vi "main.vi"() -> ()   [LabVIEW 2023]
uses:
  <vilib>/Utility/file.llb/Write Delimited Spreadsheet (DBL).vi
  <vilib>/Utility/file.llb/Read Delimited Spreadsheet (DBL).vi
  <vilib>/Instr/_visa.llb/VISA Configure Serial Port (Instr).vi
panel:
  in  "Threshold":dbl=2000.0
  in  "Open Button":bool
  in  "Save Button":bool
  out "X max":dbl
  out "X min":dbl
  out "Y max":dbl
  out "Y min":dbl
  out "Z max":dbl
  out "Z min":dbl
  out "Acc":cluster{dbl[], dbl[]}[](graph) caption="XY Graph - Dark"
  out "Z max":dbl
  out "Z min":dbl
  out "Y max":dbl
  out "Y min":dbl
  out "X min":dbl
  out "X max":dbl
  in  "Delete":bool
  out "Mag":cluster{dbl[], dbl[]}[](graph) caption="XY Graph - Dark"
  in  "Button":bool
  out "Raw Data":string
  in  "timeout (ms)":u32=100
  in  "term. char (0xA = '\\n' = LF)":u8=10 format="%.0x"
  in  "baud rate":u32=9600
  in  "COM PORT":refnum<visa-resource-name>
  # "Mag"
  # "Acc"
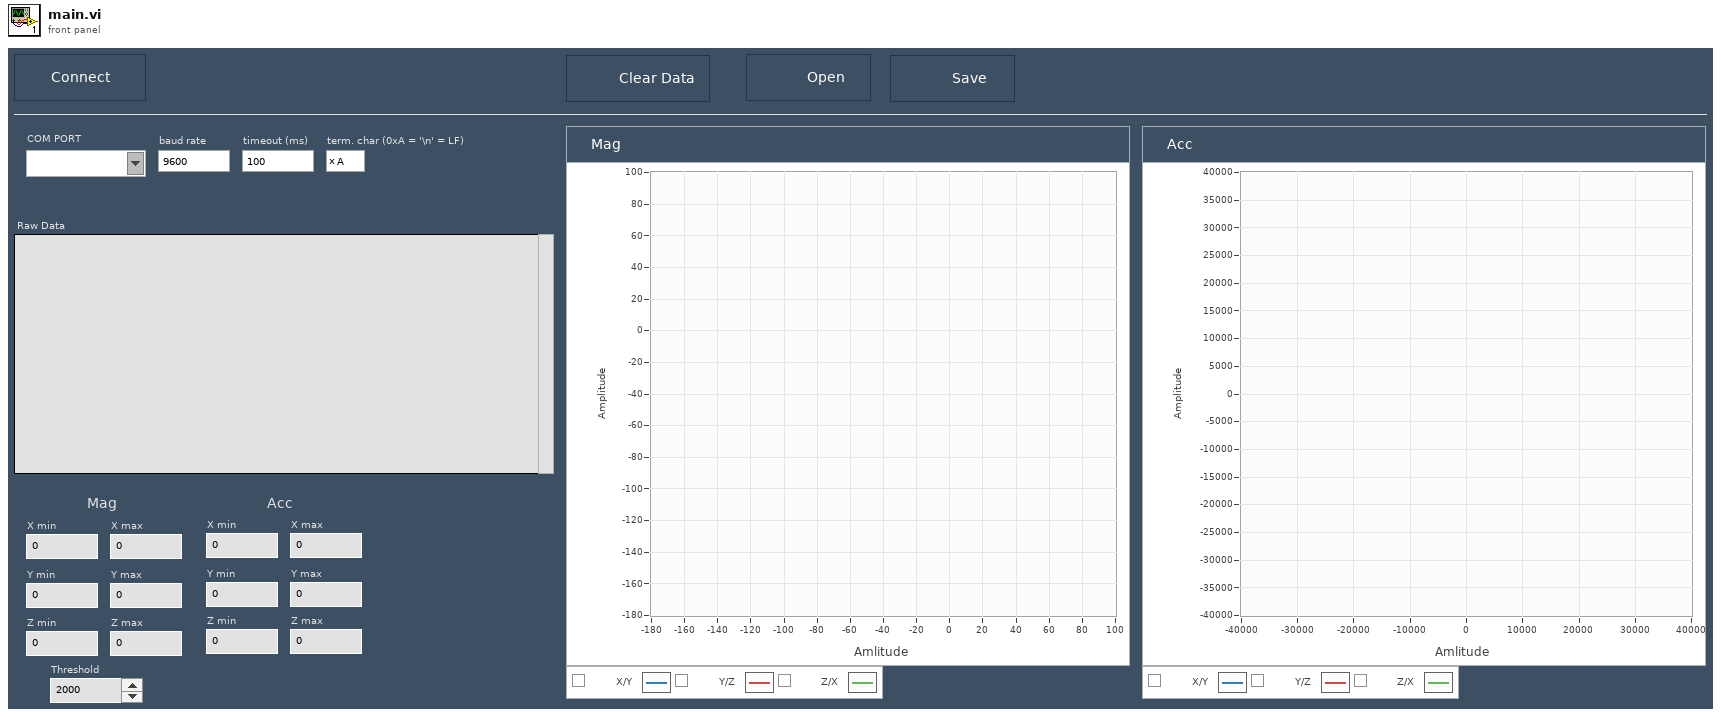
[diagram p1: front panel]
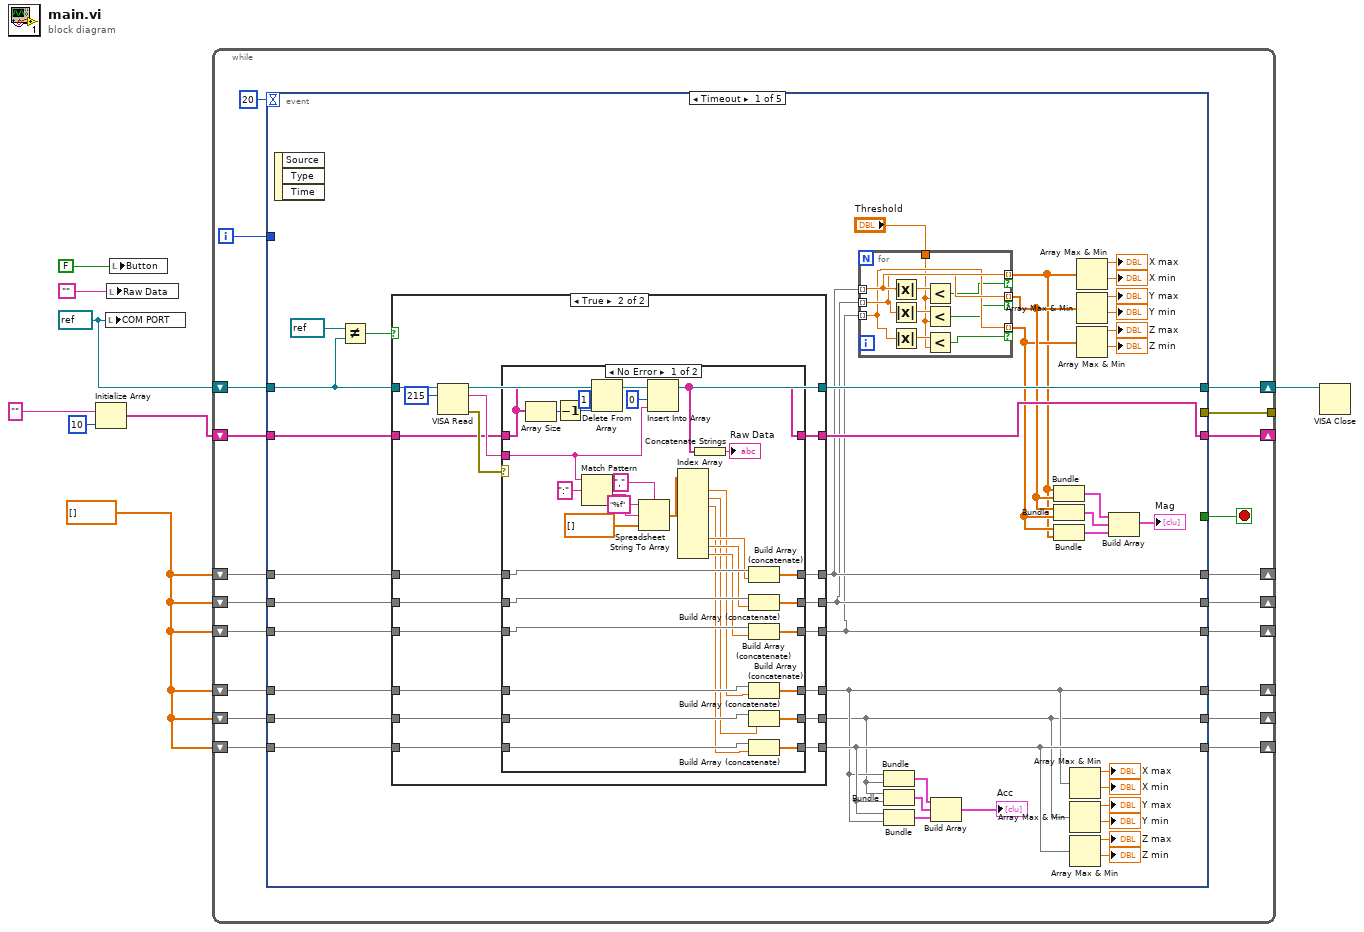
[diagram p0: block diagram]
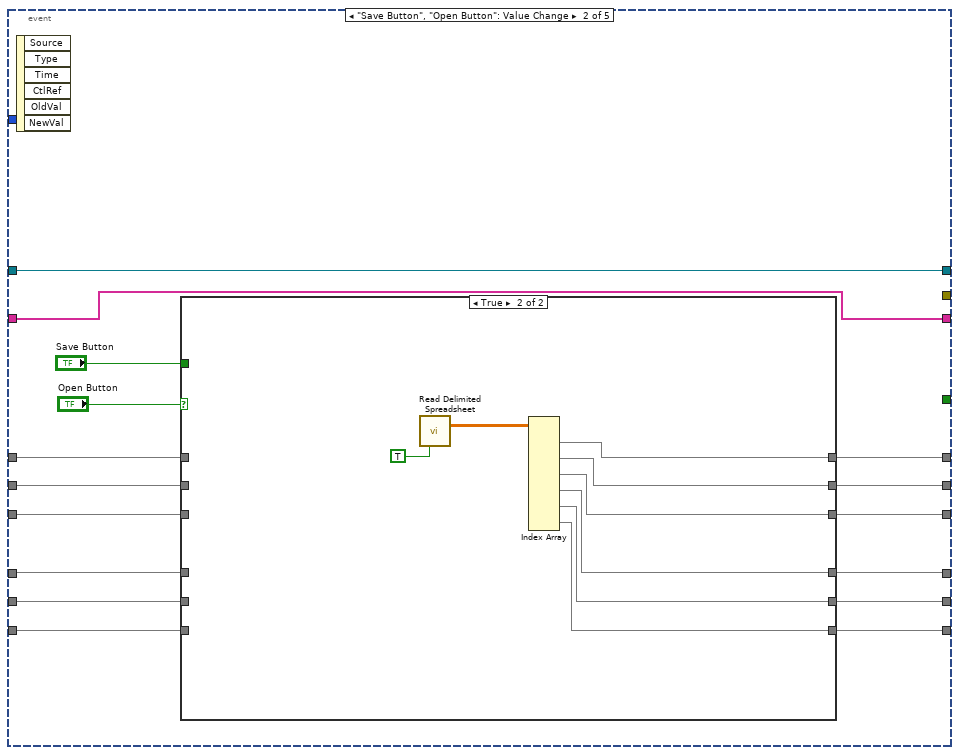
[diagram p4: hidden frame]
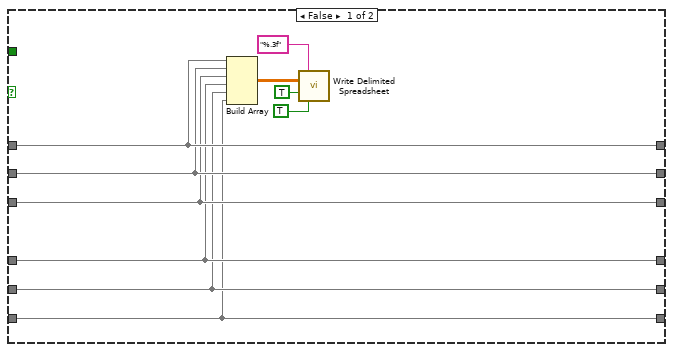
[diagram p5: hidden frame]
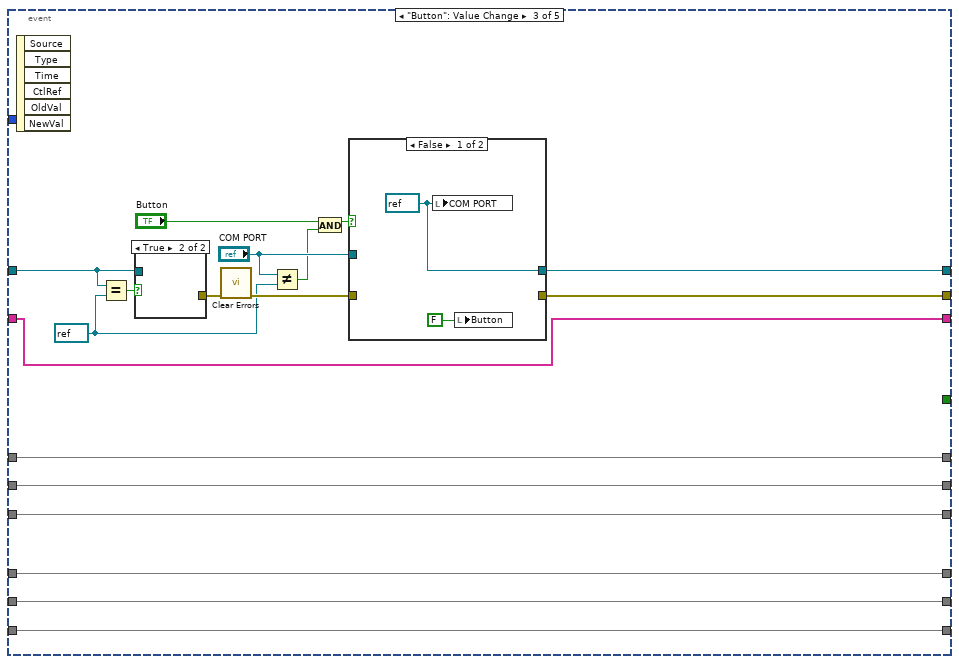
[diagram p6: hidden frame]
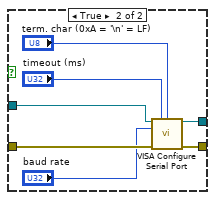
[diagram p7: hidden frame]
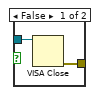
[diagram p8: hidden frame]
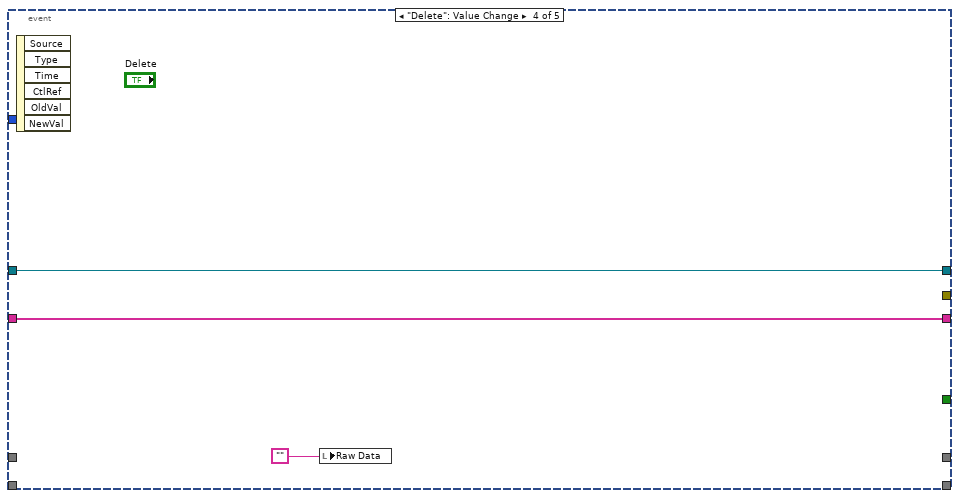
[diagram p9: hidden frame]
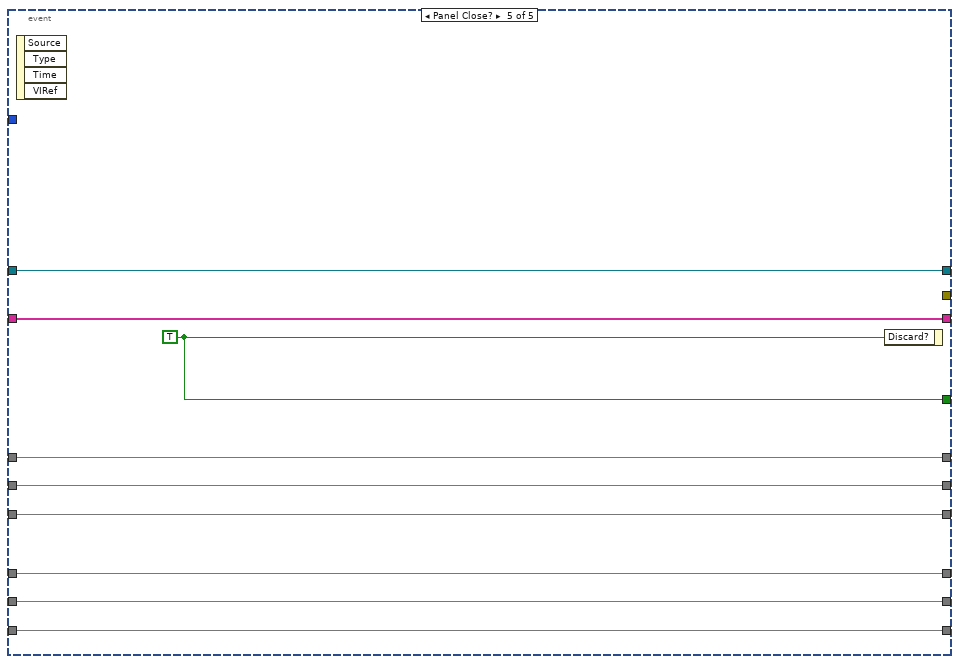
[diagram p10: hidden frame]
diagram:
  w5 = dbl[] [] ("array")
  w7 = refnum<visa-resource-name> refnum ("COM PORT")
  n1 = Initialize Array("", 10 ("dimension size")) -> (w1:string[])
  n2 = local write "COM PORT"(w7) -> ()
  n3 = local write "Raw Data"("") -> ()
  n4 = local write "Button"(FALSE ("connect")) -> ()
  n5 = while {
    tunnel: [w28] -> _
    shift-right: [w27] -> w8
    shift-left: w7 -> [w26]
    shift-right: [w23] -> _
    shift-left: w5 -> [w22]
    shift-right: [w21] -> _
    shift-left: w5 -> [w20]
    shift-right: [w19] -> _
    shift-left: w5 -> [w18]
    shift-right: [w14] -> _
    shift-left: w5 -> [w15]
    shift-right: [w13] -> _
    shift-left: w5 -> [w16]
    shift-right: [w12] -> _
    shift-left: w5 -> [w17]
    shift-right: [w10] -> _
    shift-left: w1 -> [w9]
    i -> [w11]
    stop <- w25 stop-if-true
    n6 = event shown="[0] Timeout" {
      selector: _ -> [_ _ _ _ _]
      dyn-events: _ -> [_ _ _ _ _]
      timeout: 20 -> [_ _ _ _ _]
      tunnel: [_ _ w196 _ _] -> w28
      tunnel: [w70 w163 w195 w213 w222] -> w27
      tunnel: w26 -> [w43 w163 w191 w213 w222]
      tunnel: [_ _ _ _ w221] -> w25
      tunnel: [w35 w160 w194 _ w220] -> w23
      tunnel: w22 -> [w69 w159 w194 _ w220]
      tunnel: [w34 w158 w193 _ w219] -> w21
      tunnel: w20 -> [w68 w157 w193 _ w219]
      tunnel: [w33 w155 w192 _ w218] -> w19
      tunnel: w18 -> [w67 w156 w192 _ w218]
      tunnel: w15 -> [w58 w153 w189 _ w217]
      tunnel: w16 -> [w59 w152 w188 _ w216]
      tunnel: w17 -> [w60 w149 w187 _ w215]
      tunnel: [w39 w154 w189 _ w217] -> w14
      tunnel: [w38 w151 w188 _ w216] -> w13
      tunnel: [w40 w150 w187 _ w215] -> w12
      tunnel: w11 -> [_ _ _ _ _]
      tunnel: [w37 w148 w182 w211 w214] -> w10
      tunnel: w9 -> [w36 w148 w182 w211 w214]
      event Timeout {
        n7 = event-data() -> ()  [unwired: 1 in, 3 out]
        n8 = Not Equal?(x=refnum<visa-resource-name> refnum ("COM PORT"), y=w43) -> (x != y?=w41:bool)
        n9 = case shown="True" w41 {
          tunnel: [w88 w107] -> w70
          tunnel: w43 -> [w88 w103]
          tunnel: [w87 w101] -> w35
          tunnel: w69 -> [w87 w102]
          tunnel: [w86 w100] -> w34
          tunnel: w68 -> [w86 w99]
          tunnel: [w85 w98] -> w33
          tunnel: w67 -> [w85 w97]
          tunnel: w58 -> [w84 w94]
          tunnel: w59 -> [w83 w95]
          tunnel: w60 -> [w82 w96]
          tunnel: [w84 w93] -> w39
          tunnel: [w83 w92] -> w38
          tunnel: [w82 w91] -> w40
          tunnel: [w81 w90] -> w37
          tunnel: w36 -> [w81 w89]
          frame False {
          }
          frame True {
            n10 = VISA Read(VISA resource name=w103, byte count=u32 215) -> (VISA resource name out=w107:refnum<visa-resource-name>, read buffer=w105:string, error out=w104:errorcluster)  [unwired: 1 in, 1 out]
            n11 = case shown="No Error" w104 {
              tunnel: w105 -> [w110 _]
              tunnel: w102 -> [w135 w147]
              tunnel: [w126 w147] -> w101
              tunnel: [w128 w146] -> w100
              tunnel: w99 -> [w133 w146]
              tunnel: [w127 w145] -> w98
              tunnel: w97 -> [w132 w145]
              tunnel: w94 -> [w125 w142]
              tunnel: w95 -> [w124 w143]
              tunnel: w96 -> [w123 w144]
              tunnel: [w121 w142] -> w93
              tunnel: [w122 w143] -> w92
              tunnel: [w120 w144] -> w91
              tunnel: [w109 w141] -> w90
              tunnel: w89 -> [w116 w141]
              frame No Error {
                n12 = Array Size(array=w116) -> (size(s)=w115:i32)
                n13 = Decrement(x=w115) -> (x-1=w114:i32)
                n14 = Match Pattern(string=w110, regular expression=":") -> (after substring=w138:string)  [unwired: 1 in, 3 out]
                n15 = Delete From Array(array=w116, length=1, index=w114) -> (array with subset deleted=w112:string[])  [unwired: 1 out]
                n16 = Spreadsheet String To Array(delimiter (Tab)=",", format string="%f", spreadsheet string=w138, array type (2D Dbl)=dbl[] []) -> (array=w134:dbl[])
                n17 = Insert Into Array(array=w112, index=0, new element=w110) -> (w109:string[])
                n18 = Index Array(array=w134) -> (element #1=w119:dbl, element #2=w118:dbl, element #3=w117:dbl, element #7=w131:dbl, element #8=w130:dbl, element #9=w129:dbl)  [unwired: 9 in, 3 out]
                n19 = Concatenate Strings(w109) -> (→"Raw Data":string)
                n20 = Build Array (concatenate)(w135, w131) -> (w126:dbl[])
                n21 = Build Array (concatenate)(w133, w130) -> (w128:dbl[])
                n22 = Build Array (concatenate)(w132, w129) -> (w127:dbl[])
                n23 = Build Array (concatenate)(w125, w119) -> (w121:dbl[])
                n24 = Build Array (concatenate)(w124, w118) -> (w122:dbl[])
                n25 = Build Array (concatenate)(w123, w117) -> (w120:dbl[])
              }
              frame Error {
              }
            }
          }
        }
        n26 = for {
          tunnel: w35 -> [w77] mode=indexing
          tunnel: w34 -> [w76] mode=indexing
          tunnel: w33 -> [w75] mode=indexing
          tunnel: "Threshold" -> [w74]
          tunnel: [w77] -> w29 mode=indexing if=w72
          tunnel: [w76] -> w31 mode=indexing if=w73
          tunnel: [w75] -> w30 mode=indexing if=w71
          n27 = Absolute Value(x=w77) -> (abs(x)=w80:dbl)
          n28 = Absolute Value(x=w76) -> (abs(x)=w79:dbl)
          n29 = Absolute Value(x=w75) -> (abs(x)=w78:dbl)
          n30 = Less?(x=w80, y=w74) -> (x < y?=w72:bool)
          n31 = Less?(x=w79, y=w74) -> (x < y?=w73:bool)
          n32 = Less?(x=w78, y=w74) -> (x < y?=w71:bool)
        }
        n33 = Bundle("array"=w39, "array"=w38) -> (w46:cluster{"array":dbl[], "array":dbl[]})  [unwired: 1 in]
        n34 = Bundle("array"=w38, "array"=w40) -> (w45:cluster{"array":dbl[], "array":dbl[]})  [unwired: 1 in]
        n35 = Bundle("array"=w40, "array"=w39) -> (w44:cluster{"array":dbl[], "array":dbl[]})  [unwired: 1 in]
        n36 = Build Array(w46, w45, w44) -> (→"Acc":cluster{"array":dbl[], "array":dbl[]}[])
        n37 = Bundle(w29, w31) -> (w48:cluster{dbl[], dbl[]})  [unwired: 1 in]
        n38 = Bundle(w31, w30) -> (w49:cluster{dbl[], dbl[]})  [unwired: 1 in]
        n39 = Bundle(w30, w29) -> (w50:cluster{dbl[], dbl[]})  [unwired: 1 in]
        n40 = Array Max & Min(array=w39) -> (max value=→"X max":dbl, min value=→"X min":dbl)  [unwired: 2 out]
        n41 = Array Max & Min(array=w38) -> (max value=→"Y max":dbl, min value=→"Y min":dbl)  [unwired: 2 out]
        n42 = Array Max & Min(array=w40) -> (max value=→"Z max":dbl, min value=→"Z min":dbl)  [unwired: 2 out]
        n43 = Array Max & Min(array=w29) -> (max value=→"X max":dbl, min value=→"X min":dbl)  [unwired: 2 out]
        n44 = Array Max & Min(array=w31) -> (max value=→"Y max":dbl, min value=→"Y min":dbl)  [unwired: 2 out]
        n45 = Array Max & Min(array=w30) -> (max value=→"Z max":dbl, min value=→"Z min":dbl)  [unwired: 2 out]
        n46 = Build Array(w48, w49, w50) -> (→"Mag":cluster{dbl[], dbl[]}[])
      }
      event "Save Button", "Open Button": Value Change {
        n47 = event-data() -> ()  [unwired: 1 in, 6 out]
        n48 = case shown="True" "Open Button" {
          tunnel: "Save Button" -> [_ _]
          tunnel: [w173 w179] -> w160
          tunnel: w159 -> [w173 _]
          tunnel: [w172 w178] -> w158
          tunnel: w157 -> [w172 _]
          tunnel: w156 -> [w171 _]
          tunnel: [w171 w177] -> w155
          tunnel: [w170 w176] -> w154
          tunnel: w153 -> [w170 _]
          tunnel: w152 -> [w169 _]
          tunnel: [w169 w175] -> w151
          tunnel: [w168 w174] -> w150
          tunnel: w149 -> [w168 _]
          frame False {
            n49 = Build Array(w173, w172, w171, w170, w169, w168) -> (w167:dbl[][])
            n50 = call-poly <vilib>:"Write Delimited Spreadsheet.vi"("format (%.3f)"="%.3f", "2D data"=w167, "append to file? (new file:F)"=TRUE, "transpose? (no:F)"=TRUE) -> ()  [unwired: 10 in, 2 out]
          }
          frame True {
            n51 = call-poly <vilib>:"Read Delimited Spreadsheet.vi"("transpose? (F)"=TRUE) -> ("all rows"=w180:dbl[][])  [unwired: 9 in, 5 out]
            n52 = Index Array(array=w180) -> (element #1=w179:dbl[], element #2=w178:dbl[], element #3=w177:dbl[], element #4=w176:dbl[], element #5=w175:dbl[], element #6=w174:dbl[])  [unwired: 12 in]
          }
        }
      }
      event "Button": Value Change {
        w184 = refnum<visa-resource-name> refnum ("COM PORT")
        n53 = event-data() -> ()  [unwired: 1 in, 6 out]
        n54 = Equal?(x=w191, y=w184) -> (x = y?=w199:bool)
        n55 = case shown="True" w199 {
          tunnel: w191 -> [w210 _]
          tunnel: [w209 _] -> w198
          frame False {
            n56 = VISA Close(VISA resource name=w210) -> (error out=w209:errorcluster)  [unwired: 1 in]
          }
          frame True {
          }
        }
        n57 = call <vilib>:"Clear Errors.vi"("error in (no error)"=w198) -> ("error out"=w197:errorcluster)  [unwired: 5 in, 1 out]
        n58 = Not Equal?(x="COM PORT", y=w184) -> (x != y?=w183:bool)
        n59 = And(x="Button", y=w183) -> (x .and. y?=w186:bool)
        n60 = case shown="False" w186 {
          tunnel: w197 -> [_ w208]
          tunnel: [_ w205] -> w196
          tunnel: [w201 w204] -> w195
          tunnel: "COM PORT" -> [_ w202]
          frame False {
            w201 = refnum<visa-resource-name> refnum ("COM PORT")
            n61 = local write "COM PORT"(w201) -> ()
            n62 = local write "Button"(FALSE ("connect")) -> ()
          }
          frame True {
            n63 = call-poly "VISA Configure Serial Port"("VISA resource name"=w202, "timeout (10sec)"="timeout (ms)", "termination char\n(0xA = '\\n' = LF)"="term. char (0xA = '\\n' = LF)", "baud rate (9600)"="baud rate", "error in (no error)"=w208) -> ("VISA resource name out"=w204:refnum<visa-resource-name>, "error out"=w205:errorcluster)  [unwired: 9 in]
          }
        }
      }
      event "Delete": Value Change {
        n64 = event-data() -> ()  [unwired: 1 in, 6 out]
        n65 = local write "Raw Data"("") -> ()
      }
      event Panel Close? {
        w221 = TRUE ("Discard?")
        n66 = event-data() -> ()  [unwired: 1 in, 4 out]
        n67 = event-data("Discard?"=w221) -> ()  [unwired: 1 in, 1 out]
      }
    }
  }
  n68 = VISA Close(VISA resource name=w8) -> ()  [unwired: 1 in, 1 out]
